vi "Wait on Job Completion.vi"(0 "SystemLink repo in":T3, 5 "job ID":string, 9 "timeout (ms) (10000)":u32=10000, 11 "error in (no error)":errorcluster) -> (4 "SystemLink repo out":T3, 6 "job data":T1, 10 "timed out?":bool, 15 "error out":errorcluster)   [LabVIEW 2017, in "SystemLink_Repo_API.lvlib"]
doc: "Waits until the specified job returns a status of \"succeeded\" or \"failed\".\n\nError Handling:\nOutputs Error 6000 if the job fails.\nOutputs Error 6001 if the job does not return a status of \"succeeded\" or \"failed\" within the timeout period."
uses:
  SystemLink_Repo_API.lvlib
  <vilib>/httpClient/ClientHandle.ctl
  <vilib>/httpClient/LabVIEWHTTPClient.lvlib
  systemlink repo.ctl
  syslink_job_datatype.ctl
  syslink_job.ctl
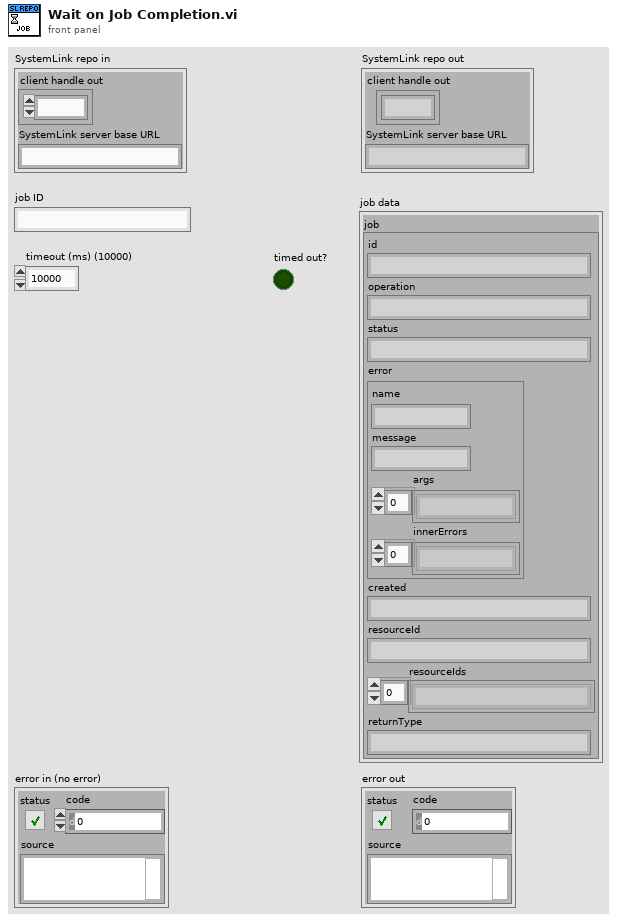
[diagram p1: front panel]
types:
  T1 = typedef "SystemLink_Repo_API.lvlib/syslink_job.ctl" = cluster{"job":T2}
  T2 = typedef "SystemLink_Repo_API.lvlib/syslink_job_datatype.ctl" = cluster{"id":string, "operation":string, "status":string, "error":cluster{"name":string, "message":string, "args":string[], "innerErrors":string[]}, "created":string, "resourceId":string, "resourceIds":string[], "returnType":string}
  T3 = typedef "SystemLink_Repo_API.lvlib/systemlink repo.ctl" = cluster{"client handle out":T4, "SystemLink server base URL":string}
  T4 = typedef "LabVIEWHTTPClient.lvlib/ClientHandle.ctl" = refnum<k1>
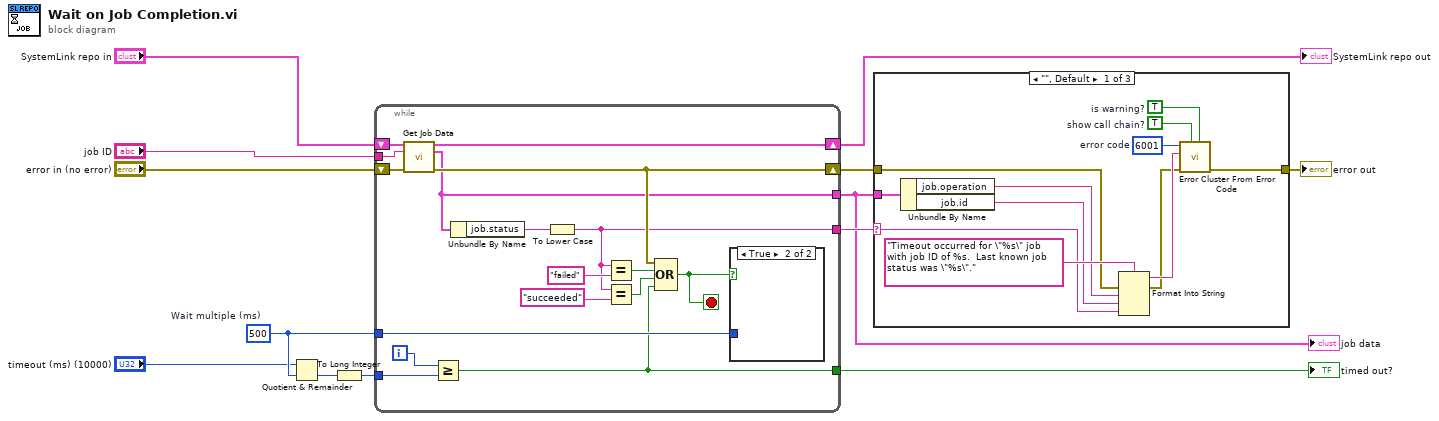
[diagram p0: block diagram]
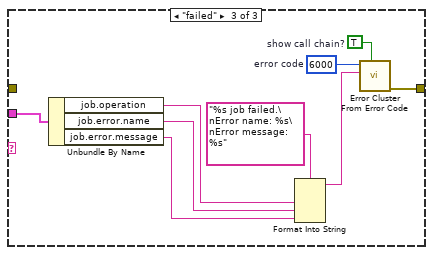
[diagram p3: hidden frame]
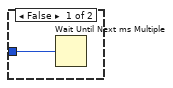
[diagram p4: hidden frame]
diagram:
  w10 = u32 500  # Wait multiple (ms)
  n1 = Quotient & Remainder(x="timeout (ms) (10000)", y=w10) -> (floor(x/y)=w11:u32)  [unwired: 1 out]
  n2 = To Long Integer(number=w11) -> (32bit integer=w12:i32)
  n3 = while {
    tunnel: "job ID" -> [w28]
    shift-right: [w25] -> w13
    shift-left: "SystemLink repo in" -> [w29]
    shift-right: [w24] -> w3
    shift-left: "error in (no error)" -> [w30]
    tunnel: w10 -> [w20]
    tunnel: w12 -> [w19]
    tunnel: [w16] -> w5
    tunnel: [w15] -> w4
    tunnel: [w14] -> w1
    i -> [w21]
    stop <- w18 stop-if-true
    n4 = call "Get Job Data.vi"("SystemLink repo in"=w29, "job ID"=w28, "error in (no error)"=w30) -> ("SystemLink repo out"=w25:T3, "job data"=w15:T1, "error out"=w24:errorcluster)  [unwired: 10 in]
    n5 = Greater Or Equal?(x=w21, y=w19) -> (x >= y?=w14:bool)
    n6 = Unbundle By Name(w15) -> ("job.status"=w17:string)
    n7 = To Lower Case(string=w17) -> (all lower case string=w16:string)
    n8 = Equal?(x=w16, y="failed") -> (x = y?=w23:bool)
    n9 = Equal?(x=w16, y="succeeded") -> (x = y?=w22:bool)
    n10 = Compound Arithmetic op=OR(w24, w23, w22, w14) -> (w18:bool)
    n11 = case shown="True" w18 {
      tunnel: w20 -> [w31 _]
      frame False {
        n12 = Wait Until Next ms Multiple(millisecond multiple=w31) -> ()  [unwired: 1 out]
      }
      frame True {
      }
    }
  }
  "SystemLink repo out" <- w13
  "timed out?" <- w1
  "job data" <- w4
  n13 = case shown="\"\", Default" w5 {
    selector: w5 -> [w32 _ _]
    tunnel: w4 -> [w43 _ w51]
    tunnel: w3 -> [w34 w44 _]
    tunnel: [w35 w44 w45] -> w2
    frame "", Default {
      w39 = TRUE  # is warning?
      w40 = 6001  # error code
      w41 = TRUE  # show call chain?
      n14 = Unbundle By Name(w43) -> ("job.operation"=w38:string, "job.id"=w37:string)
      n15 = Format Into String(format string="Timeout occurred for \"%s\" job with job ID of %s.  Last known job status was \"%s\".", error in=w34, w38, w37, w32) -> (resulting string=w36:string, error out=w33:errorcluster)  [unwired: 1 in]
      n16 = call <vilib>:"Error Cluster From Error Code.vi"("is warning? (False)"=w39, "show call chain? (False)"=w41, "error in (no error)"=w33, "error message (\"\")"=w36, "error code (0)"=w40) -> ("error out"=w35:errorcluster)  [unwired: 4 in]
    }
    frame "succeeded" {
    }
    frame "failed" {
      w46 = 6000  # error code
      w52 = TRUE  # show call chain?
      n17 = Unbundle By Name(w51) -> ("job.operation"=w50:string, "job.error.name"=w49:string, "job.error.message"=w48:string)
      n18 = Format Into String(format string="%s job failed.\nError name: %s\nError message: %s", w50, w49, w48) -> (resulting string=w47:string)  [unwired: 2 in, 1 out]
      n19 = call <vilib>:"Error Cluster From Error Code.vi"("show call chain? (False)"=w52, "error message (\"\")"=w47, "error code (0)"=w46) -> ("error out"=w45:errorcluster)  [unwired: 6 in]
    }
  }
  "error out" <- w2
